vi "String Formatting (SubVI).vi"(0 "VISA Refnum in":refnum<visa-resource-name>, 1 "Motor 6":i32, 2 "Light 1":i32, 3 "Motor 7":i32, 4 "Light 2":i32, 5 "Motor 8":i32, 6 "Motor 9":i32, 7 "error in (no error)":errorcluster, 8 "Motor 5":i32, 9 "Motor 10":i32, 10 "Motor 4":i32, 11 "Fans":i32, 12 "Motor 3":i32, 13 "Light 3":i32, 14 "Motor 2":i32, 16 "Motor 1":i32, 18 "Boolean":bool) -> (20 "VISA Refnum out":refnum<visa-resource-name>, 21 "resulting string":string, 27 "error out":errorcluster)   [LabVIEW 2019]
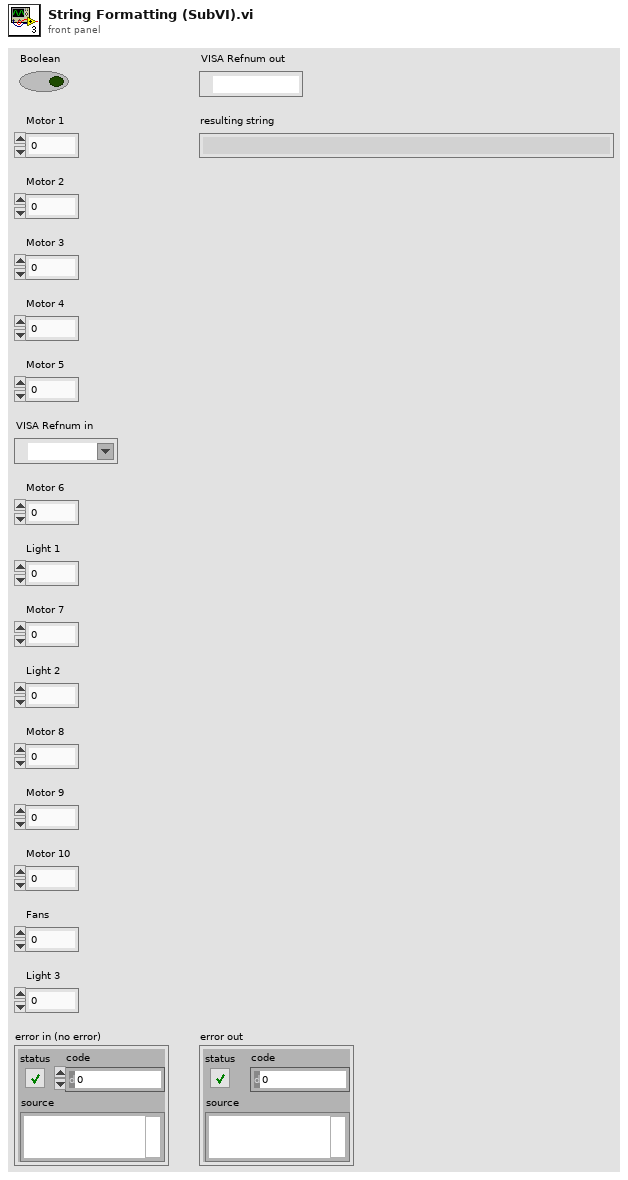
[diagram p1: front panel]
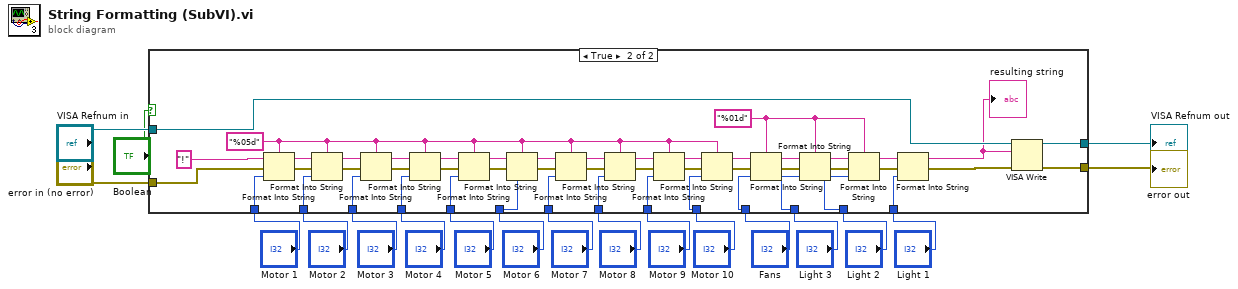
[diagram p0: block diagram]
diagram:
  n1 = case shown="True" "Boolean" {
    tunnel: "VISA Refnum in" -> [w20 w55]
    tunnel: "error in (no error)" -> [w21 w22]
    tunnel: [w20 w54] -> w4
    tunnel: [w21 w53] -> w5
    tunnel: "Motor 1" -> [_ w52]
    tunnel: "Motor 2" -> [_ w51]
    tunnel: "Motor 3" -> [_ w50]
    tunnel: "Motor 4" -> [_ w49]
    tunnel: "Motor 5" -> [_ w48]
    tunnel: "Motor 6" -> [_ w47]
    tunnel: "Motor 7" -> [_ w46]
    tunnel: "Motor 8" -> [_ w45]
    tunnel: "Motor 9" -> [_ w44]
    tunnel: "Motor 10" -> [_ w43]
    tunnel: "Fans" -> [_ w37]
    tunnel: "Light 2" -> [_ w36]
    tunnel: "Light 3" -> [_ w35]
    tunnel: "Light 1" -> [_ w27]
    frame False {
    }
    frame True {
      w28 = "%01d" ("format string")
      w38 = "%05d" ("format string")
      n2 = Format Into String(format string=w38, initial string="!" ("write buffer"), error in=w22, w52) -> (resulting string=w69:string, error out=w70:errorcluster)
      n3 = Format Into String(format string=w38, initial string=w69, error in=w70, w51) -> (resulting string=w67:string, error out=w68:errorcluster)
      n4 = Format Into String(format string=w38, initial string=w67, error in=w68, w50) -> (resulting string=w65:string, error out=w66:errorcluster)
      n5 = Format Into String(format string=w38, initial string=w65, error in=w66, w49) -> (resulting string=w63:string, error out=w64:errorcluster)
      n6 = Format Into String(format string=w38, initial string=w63, error in=w64, w48) -> (resulting string=w61:string, error out=w62:errorcluster)
      n7 = Format Into String(format string=w38, initial string=w61, error in=w62, w47) -> (resulting string=w59:string, error out=w60:errorcluster)
      n8 = Format Into String(format string=w38, initial string=w59, error in=w60, w46) -> (resulting string=w58:string, error out=w57:errorcluster)
      n9 = Format Into String(format string=w38, initial string=w58, error in=w57, w45) -> (resulting string=w40:string, error out=w42:errorcluster)
      n10 = Format Into String(format string=w38, initial string=w40, error in=w42, w44) -> (resulting string=w39:string, error out=w41:errorcluster)
      n11 = Format Into String(format string=w38, initial string=w39, error in=w41, w43) -> (resulting string=w31:string, error out=w34:errorcluster)
      n12 = Format Into String(format string=w28, initial string=w31, error in=w34, w37) -> (resulting string=w30:string, error out=w33:errorcluster)
      n13 = Format Into String(format string=w28, initial string=w30, error in=w33, w35) -> (resulting string=w29:string, error out=w32:errorcluster)
      n14 = Format Into String(format string=w28, initial string=w29, error in=w32, w36) -> (resulting string=w25:string, error out=w26:errorcluster)
      n15 = Format Into String(initial string=w25, error in=w26, w27) -> (resulting string=w23:string, error out=w24:errorcluster)  [unwired: 1 in]
      "resulting string" <- w23
      n16 = VISA Write(VISA resource name=w55, write buffer=w23, error in (no error)=w24) -> (VISA resource name out=w54:refnum<visa-resource-name>, error out=w53:errorcluster)  [unwired: 1 out]
    }
  }
  "error out" <- w5
  "VISA Refnum out" <- w4
